vi "lidar.vi"(4 "error in":errorcluster, 7 "LiDAR Configuration":string="{\n  \"type\": \"Lidar\",\n  \"listen_port\": 8200,\n  \"location\": {\n    \"x\":-10.0,\n    \"y\": 0.0,\n    \"z\":190.0\n  },\n  \"rotation\": {\n    \"pitch\":0.0,\n    \"yaw\":0.0,\n    \"roll\":0.0\n  },\n  \"max_distance\": 8000.0,\n  \"horizontal_resolution\": 0.4,\n  \"rpms\": 300.0,\n  \"n_lasers\": 32,\n  \"reset_angle\": 0.0\n}") -> (0 "error out":errorcluster, 1 "Timestamp at zero azimuth":u32, 2 "LiDAR Configuration":string, 3 "Raw data":string[](array[string]))   [LabVIEW 2019]
doc: "Configure and process the data stream for LiDAR sensor. This VI forwards the raw data to port 2368 through TCP to be visualized by VeloView."
uses:
  <vilib>/Math Plots/3D Math Plots/3D Scatter/3D Scatter Datatype/3D Scatter Datatype.lvclass
  tools/simx_common.vi
  <vilib>/Math Plots/3D Math Plots/3D Scatter/3D Scatter Datatype/Public/Plot Helper (Vector).vi
  <vilib>/Math Plots/3D Math Plots/3D Scatter/3D Scatter XCtrl/3D Scatter.xctl
  controls/Header.ctl
panel:
  out "Header":T1
  in  "Port to VeloView":u16=2368
  in  "Plot Lidar":bool
  out "Lidar Sample":refnum<class "3D Plot Datatype.lvclass">[](xcontrol)
  out "No.points":i32
  out "No.packets":i32
  out "num points":i32
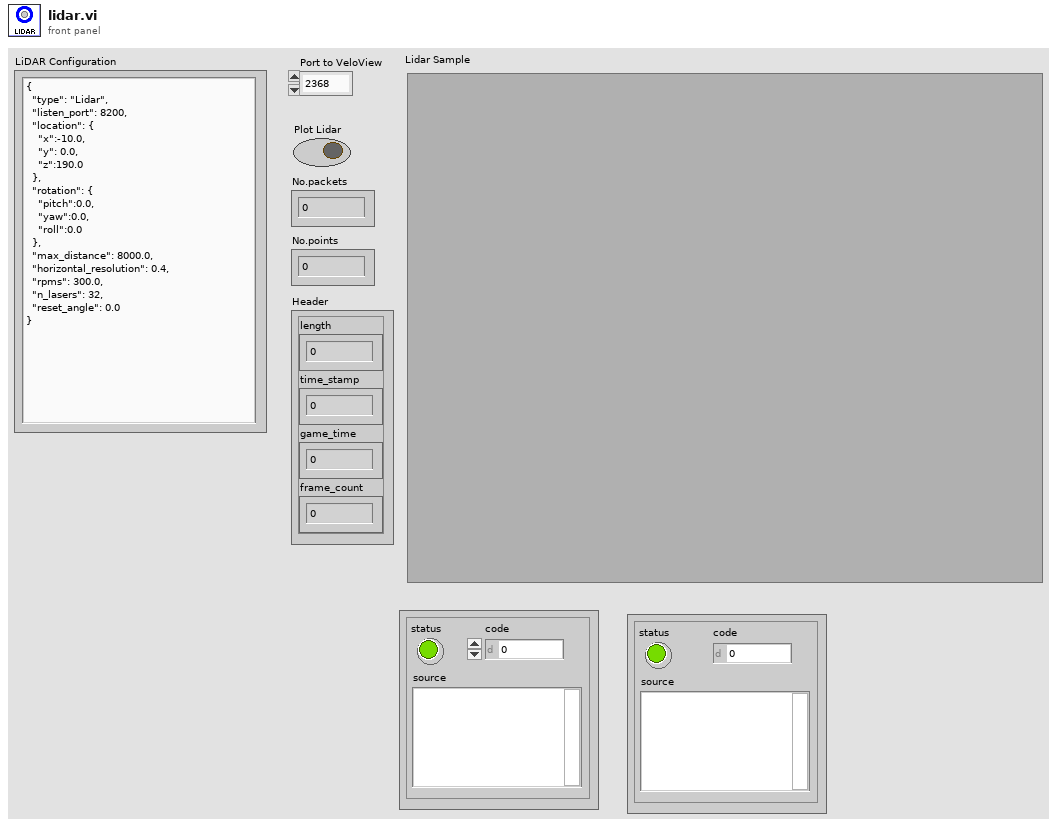
[diagram p1: front panel]
types:
  T1 = typedef "Header.ctl" = cluster{"length":u32, "time_stamp":u32, "game_time":sgl, "frame_count":u32}
  T2 = typedef "simx_connection.ctl" = cluster{"Config":T3, "Connections":T6, "Map":cluster{"lanes":cluster{"x":dbl[], "y":dbl[], "z":dbl[]}, "StartPosition":cluster{"start_points":T7, "StartRotation":dbl[], "StartLocation":dbl[]}, "Draw Map Size":T8, "DrawArea":cluster{"min_Y":dbl, "min_X":dbl, "Scale X":dbl, "Scale Y":dbl}, "Map":picture, "Map Geojson":string}}
  T3 = typedef "config.ctl" = cluster{"Trajectory":T4, "Weather":T5}
  T4 = typedef "trajectory.ctl" = cluster{"Number of frames":i32, "Frame number":i32, "Trajectory":string}
  T5 = typedef "weather.ctl" = cluster{"id":string}
  T6 = typedef "connections.ctl" = cluster{"Simulator Connection":refnum<k5>, "server_ip":string, "Port":i32, "Sensor connections":refnum<k5>[]}
  T7 = typedef "start_points.ctl" = cluster{"locations":dbl[][], "rotations":dbl[][], "type":string[]}
  T8 = typedef "LVBoundsTypeDef.ctl" = cluster{"Width":u32, "Height":u32}
  T9 = typedef "sensor_sample.ctl" = cluster{"Header":T1, "data out":string}
  T10 = cluster{"Rotational Angle (degrees)":dbl, "Vertical Angle (degrees)":dbl, "Distance (cm)":dbl, "Intensity (0-255)":u8, "Vertical Offset (cm)":dbl}[]
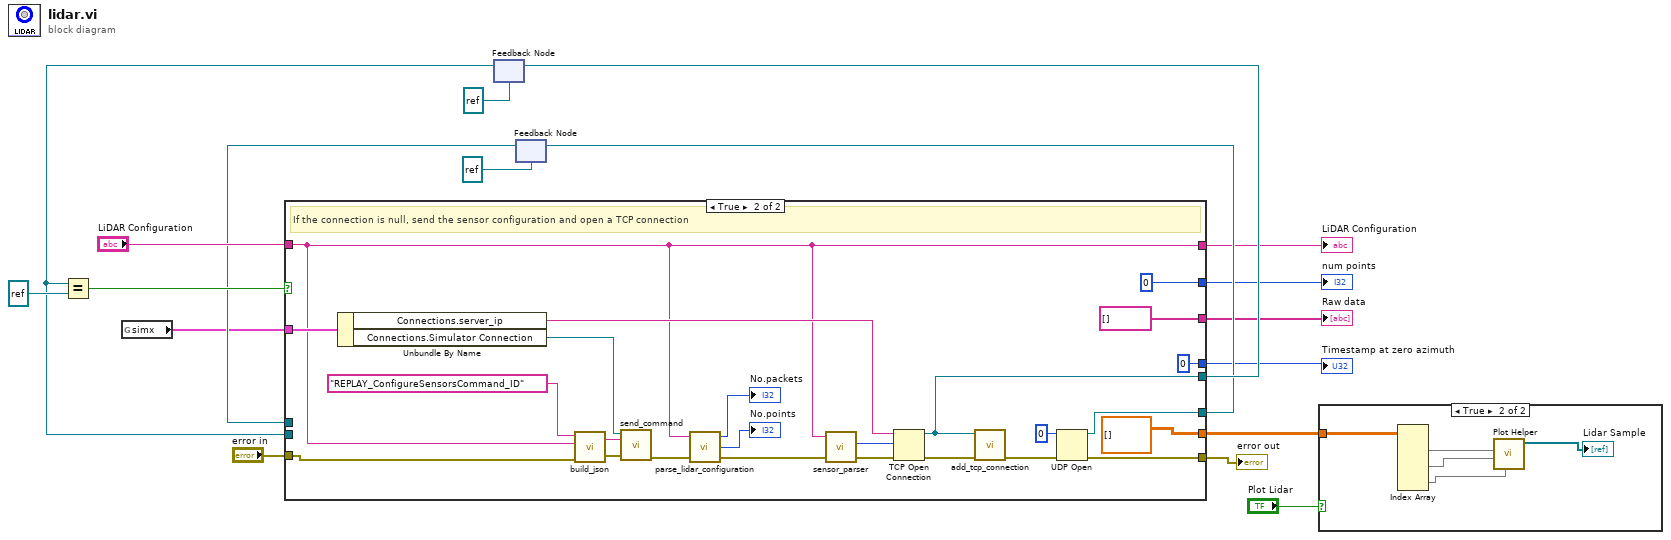
[diagram p0: block diagram]
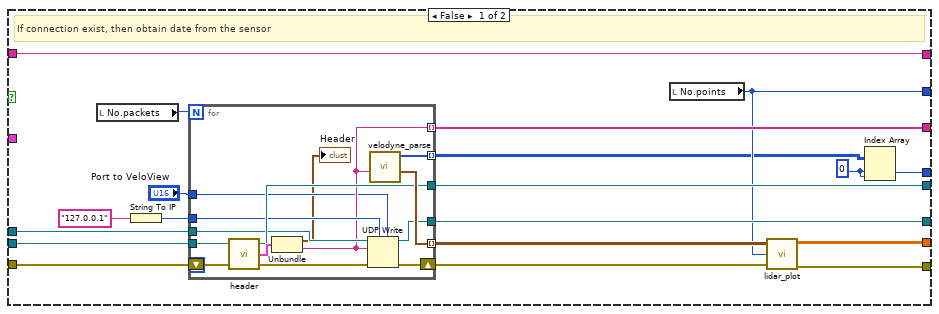
[diagram p3: hidden frame]
diagram:
  n1 = global read "simx_common.vi" "simx"() -> (w2:T2)
  n2 = feedback #1(refnum<k5> refnum ("lidar_connection")) -> (w12:refnum<k5>)
  n3 = Equal?(x=w12, y=refnum<k5> refnum ("null connection")) -> (x = y?=w14:bool)
  n4 = feedback #2(refnum<k16> refnum ("veloview_connection")) -> (w10:refnum<k16>)
  n5 = case shown="True" w14 {
    tunnel: [w35 w71] -> w18
    tunnel: "LiDAR Configuration" -> [w23 w55]
    tunnel: [w37 w61] -> w15
    tunnel: w12 -> [w36 _]
    tunnel: "error in" -> [w32 w63]
    tunnel: [w30 w72] -> w9
    tunnel: w10 -> [w31 _]
    tunnel: [w27 sgl[][] [] ("Data")] -> w4
    tunnel: [w25 string[] []] -> w7
    tunnel: [w24 0 ("No.points")] -> w6
    tunnel: [w23 w55] -> w5
    tunnel: w2 -> [_ w65]
    tunnel: [w19 u32 0 ("timestamp (us)")] -> w1
    frame False {
      w20 = 0 ("index (row)")
      # "If connection exist, then obtain date from the sensor"
      n6 = local read "No.packets"() -> (w26:i32)
      n7 = String To IP(1:"127.0.0.1" ("veloview address input")) -> (0:w28:u32)
      n8 = for {
        N: w26 -> [_]
        tunnel: w36 -> [w49]
        tunnel: [w48] -> w34 mode=indexing
        tunnel: [w47] -> w37
        shift-right: [w42] -> w33
        shift-left: w32 -> [w50]
        tunnel: w31 -> [w46]
        tunnel: [w45] -> w30
        tunnel: w28 -> [w44]
        tunnel: [w40] -> w25 mode=indexing
        tunnel: [w41] -> w21 mode=indexing
        tunnel: "Port to VeloView" -> [w39]
        n9 = call "header.vi"("error in"=w50, "TCP Network Connection in"=w49) -> ("error out"=w43:errorcluster, "Sensor sample"=w51:T9, "TCP Network Connection out"=w47:refnum<k5>)  [unwired: 1 in]
        n10 = Unbundle(w51) -> ("Header"=→"Header":T1, "data out"=w40:string)
        n11 = UDP Write(address=w44, port or service name=w39, connection ID=w46, data in=w40, 8:w43) -> (error out=w42:errorcluster, 3:w45:refnum<k16>)  [unwired: 1 in]
        n12 = call "velodyne_parse.vi"("Raw LiDAR data"=w40) -> ("Pased LIDAR Data"=w48:T10, "Timestamps"=w41:u32[])  [unwired: 5 in]
      }
      n13 = local read "No.points"() -> (w24:i32)
      n14 = call "lidar_plot.vi"("LiDAR Data"=w34, "Number points"=w24, "error in"=w33) -> ("LiDAR points"=w27:sgl[][], "error out"=w35:errorcluster)  [unwired: 1 in, 1 out]
      n15 = Index Array(array=w21, index (row)=w20, index (col)=w20) -> (element=w19:u32)
    }
    frame True {
      # "If the connection is null, send the sensor configuration and open a TCP connection"
      n16 = Unbundle By Name(w65) -> ("Connections.server_ip"=w64:string, "Connections.Simulator Connection"=w60:refnum<k5>)
      n17 = call "build_json.vi"("error in"=w63, "Message"=w55, "Command_ID"="REPLAY_ConfigureSensorsCommand_ID") -> ("error out"=w73:errorcluster, "JSON Out"=w74:string)  [unwired: 1 in]
      n18 = call "send_command.vi"("error in"=w73, "JSON Command"=w74, "TCP Network Connection in"=w60) -> ("error out"=w58:errorcluster)  [unwired: 1 in, 3 out]
      n19 = call "parse_lidar_configuration.vi"("error in"=w58, "Lidar configuration"=w55) -> ("error out"=w57:errorcluster, "Number points"=→"No.points":i32, "Number packets"=→"No.packets":i32)  [unwired: 1 in]
      n20 = call "sensor_parser.vi"("Sensor configuration"=w55, "error in"=w57) -> ("Port out"=w54:u16, "error out"=w56:errorcluster)  [unwired: 1 in, 2 out]
      n21 = TCP Open Connection(address=w64, remote port or service name=w54, error in (no error)=w56) -> (connection ID=w61:refnum<k5>, error out=w69:errorcluster)  [unwired: 2 in]
      n22 = call "add_tcp_connection.vi"("error in"=w69, "Sensor connection"=w61) -> ("error out"=w62:errorcluster)  [unwired: 5 in]
      n23 = UDP Open(8:w62, 11:u16 0 ("local veloview tx port")) -> (port=w72:refnum<k16>, 0:w71:errorcluster)  [unwired: 3 in, 1 out]
    }
  }
  "error out" <- w18
  "Raw data" <- w7
  "num points" <- w6
  "LiDAR Configuration" <- w5
  "Timestamp at zero azimuth" <- w1
  n24 = feedback-in #1(w15) -> ()
  n25 = feedback-in #2(w9) -> ()
  n26 = case shown="True" "Plot Lidar" {
    tunnel: w4 -> [_ w79]
    frame False {
    }
    frame True {
      n27 = Index Array(array=w79) -> (element #1=w78:sgl[], element #2=w77:sgl[], element #3=w76:sgl[])  [unwired: 6 in]
      n28 = call-poly <vilib>:"Plot Helper.vi"("z vector"=w76, "y vector"=w77, "x vector"=w78) -> ("3D Plot lvclass Array out"=→"Lidar Sample":refnum<class "3D Plot Datatype.lvclass">[])  [unwired: 3 in, 5 out]
    }
  }
